vi "FTW-Actor-ConfigureTiming-Reactor.vi"(0 "FTW Actor Instance":refnum<class "FTW-Actor-Instance.lvclass">, 11 "error in":errorcluster) -> (4 "FTW Actor Instance out":refnum<class "FTW-Actor-Instance.lvclass">, 15 "error out":errorcluster)   [LabVIEW 2015, in "FTW-Actor-Instance.lvclass"]
uses:
  FTW-Actor-Instance.lvclass
panel:
  # "Inputs"
  # "Outputs"
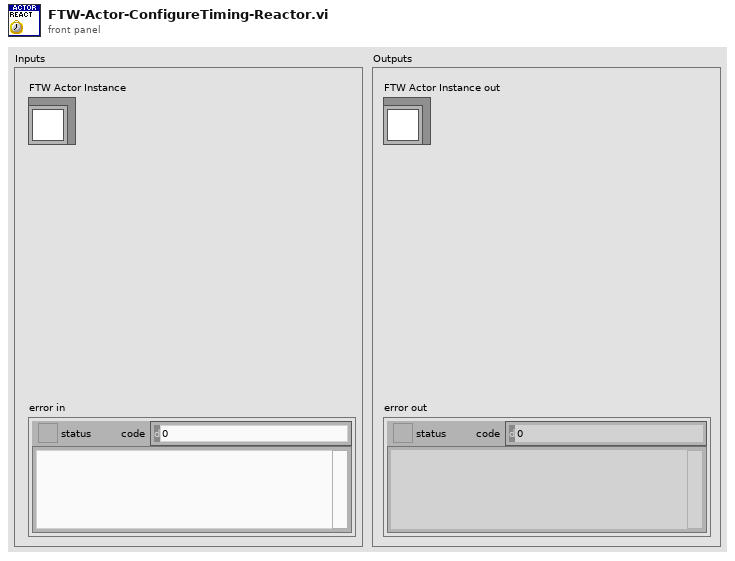
[diagram p1: front panel]
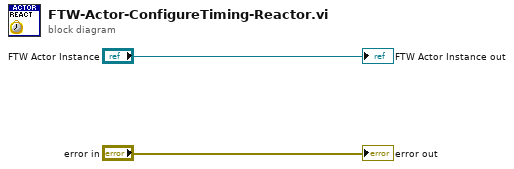
[diagram p0: block diagram]
diagram:
  "error out" <- "error in"
  "FTW Actor Instance out" <- "FTW Actor Instance"
